vi "ELVIS III v1.0 AI Block Read Bank A.vi"(6 "CNT":u8, 7 "Bank Config":u8[](array[numeric]), 8 "error in (no error)":errorcluster, 9 "Count (tick/s)":u32, 10 "Number of Samples":u32=1000, 11 "AI Block Channels FPGA Reference":T1) -> (0 "error out":errorcluster, 3 "Data":dbl[][](array[numeric]))   [LabVIEW 2021]
uses:
  <vilib>/myRIO/Common/Instrument Driver Framework/ELVIS III v1.0/AI Block/typedefs/ELVIS III AI Block Channels FPGA Reference.ctl
  <vilib>/Utility/error.llb/Error Cluster From Error Code.vi
  <vilib>/rvi/errors/niLvFpgaAdjustHostInterfaceError.vi
  <vilib>/rvi/interface/nirviReadWriteControl/nirviReadWriteControl.xnode
  <vilib>/rvi/interface/nirviMethod/nirviMethod.xnode
  <vilib>/rvi/interface/Simulation/niFpgaSimulationCallBeginRW.vi
  <vilib>/rvi/errors/niLvFpgaMergeErrorWithErrorCode.vi
  NiFpgaLv.dll
  <vilib>/FPGAPlugInAG/Dynamic/niLvFpga_StartFifo_Dynamic.vi
  <vilib>/FPGAPlugInAG/Dynamic/niLvFpga_StopFifo_Dynamic.vi
  <vilib>/FPGAPlugInAG/Dynamic/niLvFpga_ReadFifo_Dynamic.vi
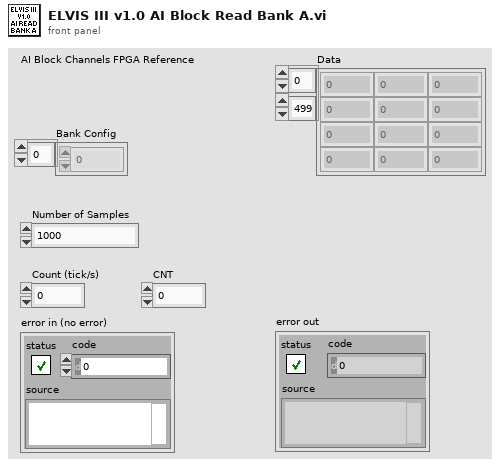
[diagram p1: front panel]
types:
  T1 = typedef "ELVIS III AI Block Channels FPGA Reference.ctl" = refnum<k20>
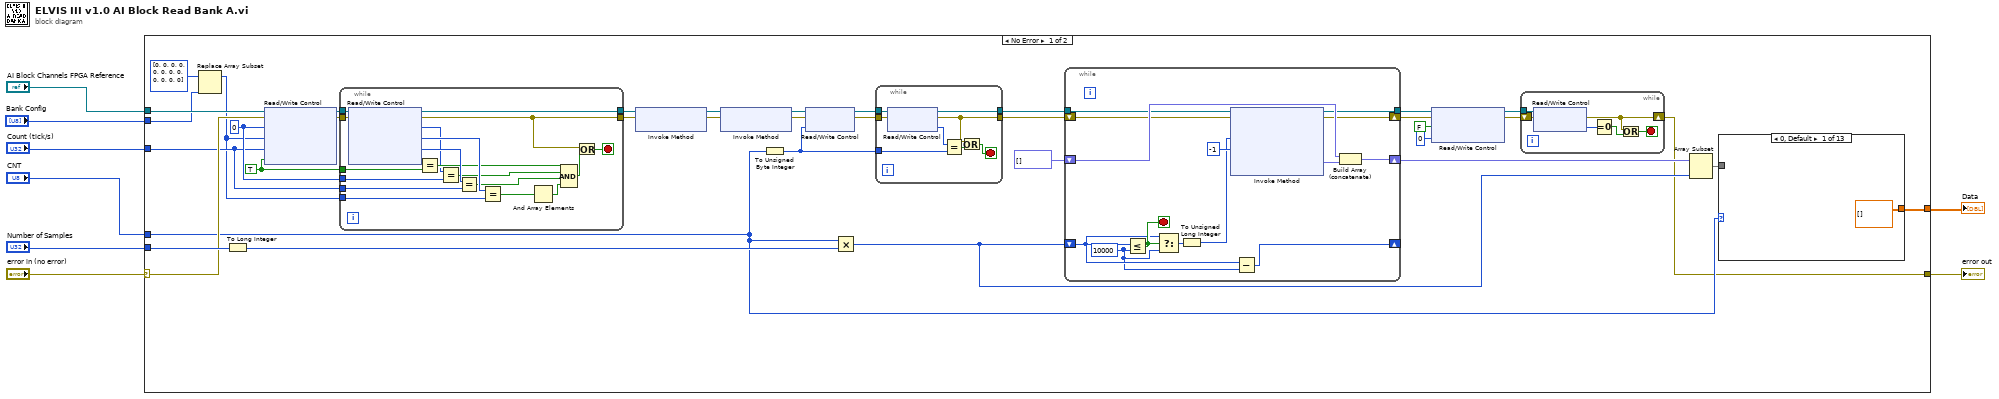
[diagram p0: block diagram]
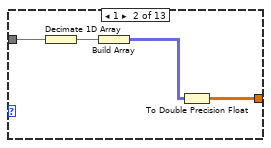
[diagram p2: hidden frame]
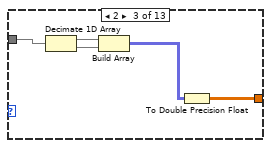
[diagram p3: hidden frame]
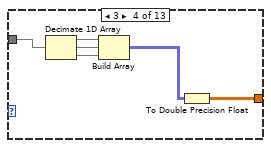
[diagram p4: hidden frame]
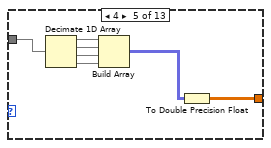
[diagram p5: hidden frame]
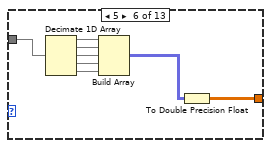
[diagram p6: hidden frame]
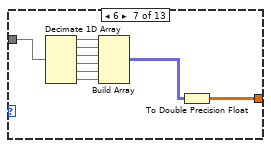
[diagram p7: hidden frame]
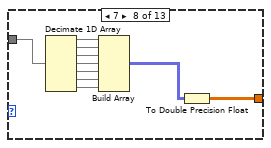
[diagram p8: hidden frame]
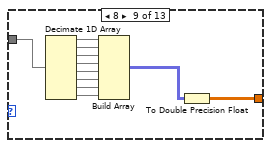
[diagram p9: hidden frame]
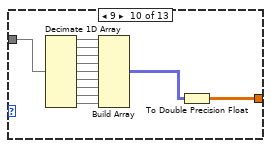
[diagram p10: hidden frame]
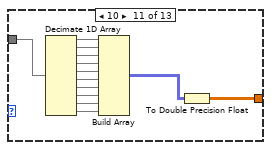
[diagram p11: hidden frame]
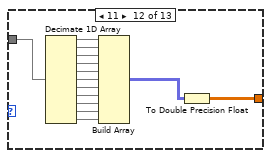
[diagram p12: hidden frame]
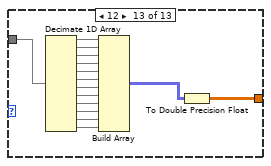
[diagram p13: hidden frame]
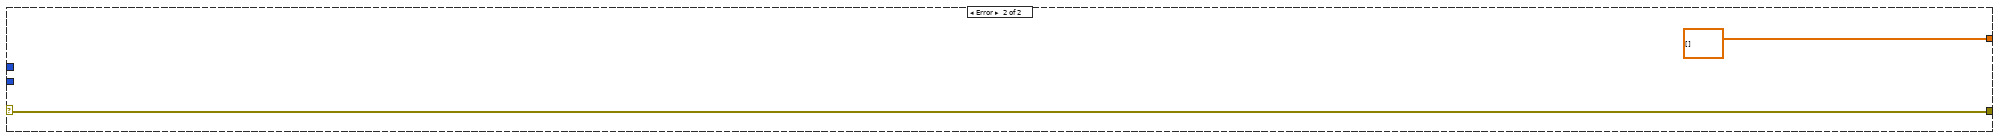
[diagram p14: hidden frame]
diagram:
  n1 = case shown="No Error" "error in (no error)" {
    selector: "error in (no error)" -> [w18 w207]
    tunnel: "AI Block Channels FPGA Reference" -> [w44 _]
    tunnel: "Count (tick/s)" -> [w17 _]
    tunnel: "Number of Samples" -> [w20 _]
    tunnel: "Bank Config" -> [w21 _]
    tunnel: [w28 dbl[][] [] ("Data")] -> w3
    tunnel: [w10 w207] -> w2
    tunnel: "CNT" -> [w13 _]
    frame No Error {
      w26 = TRUE ("AI.A.DMA_ENA")
      w23 = u8 0 ("AI.A.CNT")
      n2 = Replace Array Subset(array=u8[] [0, 0, 0, 0, 0, 0, 0, 0, 0, 0, 0, 0] ("AI.A.CNFG"), new element=w21) -> (w16:u8[])  [unwired: 1 in]
      n3 = To Long Integer(number=w20) -> (32bit integer=w19:i32)
      n4 = xnode "Read/Write Control"("FPGA VI Reference In"=w44, "error in"=w18, "AI.A.CNT"=w23, "AI.A.CNFG"=w16, "AI.A.CNTR"=w17, "AI.A.DMA_ENA"=w26) -> ("FPGA VI Reference Out"=w42:T1, "error out"=w43:errorcluster)
      n5 = while {
        tunnel: w42 -> [w206]
        tunnel: w43 -> [w205]
        tunnel: [w204] -> w39
        tunnel: [w196] -> w38
        tunnel: w16 -> [w194]
        tunnel: w17 -> [w202]
        tunnel: w23 -> [w200]
        tunnel: w26 -> [w191]
        stop <- w195 stop-if-true
        n6 = xnode "Read/Write Control"("FPGA VI Reference In"=w206, "error in"=w205) -> ("FPGA VI Reference Out"=w204:T1, "error out"=w196:errorcluster, "AI.A.CNT"=w189:u8, "AI.A.CNFG"=w203:u8[], "AI.A.CNTR"=w201:u32, "AI.A.DMA_ENA"=w192:bool)
        n7 = Equal?(x=w192, y=w191) -> (x = y?=w190:bool)
        n8 = Equal?(x=w189, y=w200) -> (x = y?=w199:bool)
        n9 = Equal?(x=w201, y=w202) -> (x = y?=w198:bool)
        n10 = Equal?(x=w203, y=w194) -> (x = y?=w188:bool[])
        n11 = And Array Elements(Boolean array=w188) -> (logical AND=w193:bool)
        n12 = Compound Arithmetic op=AND(w190, w199, w198, w193) -> (w197:bool)
        n13 = Or(x=w196, y=w197) -> (x .or. y?=w195:bool)
      }
      n14 = xnode "Invoke Method"("FPGA VI Reference In"=w39, "error in"=w38) -> ("FPGA VI Reference Out"=w41:T1, "error out"=w40:errorcluster)
      n15 = xnode "Invoke Method"("FPGA VI Reference In"=w41, "error in"=w40) -> ("FPGA VI Reference Out"=w35:T1, "error out"=w34:errorcluster)
      n16 = To Unsigned Byte Integer(number=w13) -> (unsigned 8bit integer=w27:u8)
      n17 = xnode "Read/Write Control"("FPGA VI Reference In"=w35, "error in"=w34, "AI.A.CNT"=w27) -> ("FPGA VI Reference Out"=w32:T1, "error out"=w33:errorcluster)
      n18 = Multiply(x=w13, y=w19) -> (x*y=w15:i32)
      n19 = while {
        tunnel: w33 -> [w173]
        tunnel: w32 -> [w172]
        tunnel: [w168] -> w30
        tunnel: [w171] -> w31
        tunnel: w27 -> [w169]
        stop <- w166 stop-if-true
        n20 = xnode "Read/Write Control"("FPGA VI Reference In"=w172, "error in"=w173) -> ("FPGA VI Reference Out"=w171:T1, "error out"=w168:errorcluster, "AI.A.CNT"=w170:u8)
        n21 = Equal?(x=w170, y=w169) -> (x = y?=w167:bool)
        n22 = Or(x=w168, y=w167) -> (x .or. y?=w166:bool)
      }
      n23 = while {
        tunnel: w31 -> [w177]
        shift-right: [w175] -> w24
        shift-left: w30 -> [w174]
        shift-right: [w180] -> w36
        shift-left: fxp<+/-,24,5>[] [] ("Data") -> [w181]
        shift-right: [w183] -> _
        shift-left: w15 -> [w185]
        tunnel: [w176] -> w14
        stop <- w186 stop-if-true
        w184 = 10000 ("y")
        n24 = Less Or Equal?(x=w185, y=w184) -> (x <= y?=w186:bool)
        n25 = Select(t=w185, s=w186, f=w184) -> (s? t:f=w179:i32)
        n26 = To Unsigned Long Integer(number=w179) -> (unsigned 32bit integer=w178:u32)
        n27 = xnode "Invoke Method"("FPGA VI Reference In"=w177, "error in"=w174, "Number of Elements"=w178, "Timeout (ms)"=-1) -> ("FPGA VI Reference Out"=w176:T1, "error out"=w175:errorcluster, "Data"=w182:fxp<+/-,24,5>[])  [unwired: 1 out]
        n28 = Subtract(x=w185, y=w184) -> (x-y=w183:i32)
        n29 = Build Array (concatenate)(w181, w182) -> (w180:fxp<+/-,24,5>[])
      }
      n30 = xnode "Read/Write Control"("FPGA VI Reference In"=w14, "error in"=w24, "AI.A.DMA_ENA"=FALSE ("Flag"), "AI.A.CNT"=u8 0) -> ("FPGA VI Reference Out"=w11:T1, "error out"=w9:errorcluster)
      n31 = while {
        tunnel: w11 -> [w50]
        shift-right: [w48] -> w10
        shift-left: w9 -> [w45]
        stop <- w46 stop-if-true
        n32 = xnode "Read/Write Control"("FPGA VI Reference In"=w50, "error in"=w45) -> ("error out"=w48:errorcluster, "AI.A.STAT"=w49:u8)  [unwired: 1 out]
        n33 = Equal To 0?(x=w49) -> (x = 0?=w47:bool)
        n34 = Or(x=w48, y=w47) -> (x .or. y?=w46:bool)
      }
      n35 = Array Subset(array=w36, length=w15) -> (w29:fxp<+/-,24,5>[])  [unwired: 1 in]
      n36 = case shown="0, Default" w13 {
        tunnel: w29 -> [_ w55 w60 w66 w73 w81 w90 w100 w111 w123 w136 w150 w165]
        tunnel: [dbl[][] [] w53 w58 w64 w71 w79 w88 w98 w109 w121 w134 w148 w163] -> w28
        frame 0, Default {
        }
        frame 1 {
          n37 = Decimate 1D Array(w55) -> (w54:fxp<+/-,24,5>[])
          n38 = Build Array(w54) -> (w52:fxp<+/-,24,5>[][])
          n39 = To Double Precision Float(number=w52) -> (double precision float=w53:dbl[][])
        }
        frame 2 {
          n40 = Decimate 1D Array(w60) -> (w59:fxp<+/-,24,5>[], w56:fxp<+/-,24,5>[])
          n41 = Build Array(w59, w56) -> (w57:fxp<+/-,24,5>[][])
          n42 = To Double Precision Float(number=w57) -> (double precision float=w58:dbl[][])
        }
        frame 3 {
          n43 = Decimate 1D Array(w66) -> (w65:fxp<+/-,24,5>[], w62:fxp<+/-,24,5>[], w61:fxp<+/-,24,5>[])
          n44 = Build Array(w65, w62, w61) -> (w63:fxp<+/-,24,5>[][])
          n45 = To Double Precision Float(number=w63) -> (double precision float=w64:dbl[][])
        }
        frame 4 {
          n46 = Decimate 1D Array(w73) -> (w72:fxp<+/-,24,5>[], w69:fxp<+/-,24,5>[], w68:fxp<+/-,24,5>[], w67:fxp<+/-,24,5>[])
          n47 = Build Array(w72, w69, w68, w67) -> (w70:fxp<+/-,24,5>[][])
          n48 = To Double Precision Float(number=w70) -> (double precision float=w71:dbl[][])
        }
        frame 5 {
          n49 = Decimate 1D Array(w81) -> (w80:fxp<+/-,24,5>[], w77:fxp<+/-,24,5>[], w76:fxp<+/-,24,5>[], w75:fxp<+/-,24,5>[], w74:fxp<+/-,24,5>[])
          n50 = Build Array(w80, w77, w76, w75, w74) -> (w78:fxp<+/-,24,5>[][])
          n51 = To Double Precision Float(number=w78) -> (double precision float=w79:dbl[][])
        }
        frame 6 {
          n52 = Decimate 1D Array(w90) -> (w89:fxp<+/-,24,5>[], w86:fxp<+/-,24,5>[], w85:fxp<+/-,24,5>[], w84:fxp<+/-,24,5>[], w83:fxp<+/-,24,5>[], w82:fxp<+/-,24,5>[])
          n53 = Build Array(w89, w86, w85, w84, w83, w82) -> (w87:fxp<+/-,24,5>[][])
          n54 = To Double Precision Float(number=w87) -> (double precision float=w88:dbl[][])
        }
        frame 7 {
          n55 = Decimate 1D Array(w100) -> (w99:fxp<+/-,24,5>[], w96:fxp<+/-,24,5>[], w95:fxp<+/-,24,5>[], w94:fxp<+/-,24,5>[], w93:fxp<+/-,24,5>[], w92:fxp<+/-,24,5>[], w91:fxp<+/-,24,5>[])
          n56 = Build Array(w99, w96, w95, w94, w93, w92, w91) -> (w97:fxp<+/-,24,5>[][])
          n57 = To Double Precision Float(number=w97) -> (double precision float=w98:dbl[][])
        }
        frame 8 {
          n58 = Decimate 1D Array(w111) -> (w110:fxp<+/-,24,5>[], w107:fxp<+/-,24,5>[], w106:fxp<+/-,24,5>[], w105:fxp<+/-,24,5>[], w104:fxp<+/-,24,5>[], w103:fxp<+/-,24,5>[], w102:fxp<+/-,24,5>[], w101:fxp<+/-,24,5>[])
          n59 = Build Array(w110, w107, w106, w105, w104, w103, w102, w101) -> (w108:fxp<+/-,24,5>[][])
          n60 = To Double Precision Float(number=w108) -> (double precision float=w109:dbl[][])
        }
        frame 9 {
          n61 = Decimate 1D Array(w123) -> (w122:fxp<+/-,24,5>[], w119:fxp<+/-,24,5>[], w118:fxp<+/-,24,5>[], w117:fxp<+/-,24,5>[], w116:fxp<+/-,24,5>[], w115:fxp<+/-,24,5>[], w114:fxp<+/-,24,5>[], w113:fxp<+/-,24,5>[], w112:fxp<+/-,24,5>[])
          n62 = Build Array(w122, w119, w118, w117, w116, w115, w114, w113, w112) -> (w120:fxp<+/-,24,5>[][])
          n63 = To Double Precision Float(number=w120) -> (double precision float=w121:dbl[][])
        }
        frame 10 {
          n64 = Decimate 1D Array(w136) -> (w135:fxp<+/-,24,5>[], w132:fxp<+/-,24,5>[], w131:fxp<+/-,24,5>[], w130:fxp<+/-,24,5>[], w129:fxp<+/-,24,5>[], w128:fxp<+/-,24,5>[], w127:fxp<+/-,24,5>[], w126:fxp<+/-,24,5>[], w125:fxp<+/-,24,5>[], w124:fxp<+/-,24,5>[])
          n65 = Build Array(w135, w132, w131, w130, w129, w128, w127, w126, w125, w124) -> (w133:fxp<+/-,24,5>[][])
          n66 = To Double Precision Float(number=w133) -> (double precision float=w134:dbl[][])
        }
        frame 11 {
          n67 = Decimate 1D Array(w150) -> (w149:fxp<+/-,24,5>[], w146:fxp<+/-,24,5>[], w145:fxp<+/-,24,5>[], w144:fxp<+/-,24,5>[], w143:fxp<+/-,24,5>[], w142:fxp<+/-,24,5>[], w141:fxp<+/-,24,5>[], w140:fxp<+/-,24,5>[], w139:fxp<+/-,24,5>[], w138:fxp<+/-,24,5>[], w137:fxp<+/-,24,5>[])
          n68 = Build Array(w149, w146, w145, w144, w143, w142, w141, w140, w139, w138, w137) -> (w147:fxp<+/-,24,5>[][])
          n69 = To Double Precision Float(number=w147) -> (double precision float=w148:dbl[][])
        }
        frame 12 {
          n70 = Decimate 1D Array(w165) -> (w164:fxp<+/-,24,5>[], w161:fxp<+/-,24,5>[], w160:fxp<+/-,24,5>[], w159:fxp<+/-,24,5>[], w158:fxp<+/-,24,5>[], w157:fxp<+/-,24,5>[], w156:fxp<+/-,24,5>[], w155:fxp<+/-,24,5>[], w154:fxp<+/-,24,5>[], w153:fxp<+/-,24,5>[], w152:fxp<+/-,24,5>[], w151:fxp<+/-,24,5>[])
          n71 = Build Array(w164, w161, w160, w159, w158, w157, w156, w155, w154, w153, w152, w151) -> (w162:fxp<+/-,24,5>[][])
          n72 = To Double Precision Float(number=w162) -> (double precision float=w163:dbl[][])
        }
      }
    }
    frame Error {
    }
  }
  "error out" <- w2
  "Data" <- w3
